vi "background worker.vi"(11 "connection maintainer in":refnum<class "connection maintainer.lvclass">) -> ()   [LabVIEW 2015, in "connection maintainer.lvclass"]
uses:
  connection maintainer.lvclass
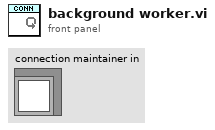
[diagram p1: front panel]
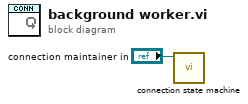
[diagram p0: block diagram]
diagram:
  n1 = call "connection state machine.vi"("connection in"="connection maintainer in") -> ()  [unwired: 11 in]
